vi "Add.vi"() -> ()   [LabVIEW 2025]
panel:
  in  "B":dbl
  in  "A":dbl
  out "C":dbl
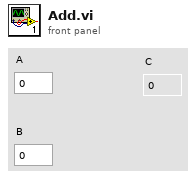
[diagram p1: front panel]
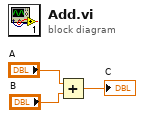
[diagram p0: block diagram]
diagram:
  n1 = Add(x="A", y="B") -> (x+y=→"C":dbl)
